vi "rma.vi"() -> ()   [LabVIEW 2016]
panel:
  out "new picture":picture
  out "Waveform Chart":cluster{"xpp":dbl, "SP":dbl}(graph)
  in  "Stop Button":bool
  in  "Ki":dbl
  in  "KD":dbl
  in  "kP":dbl
  in  "SP":dbl
  in  "F":dbl
  in  "k":dbl
  in  "b":dbl
  in  "m":dbl
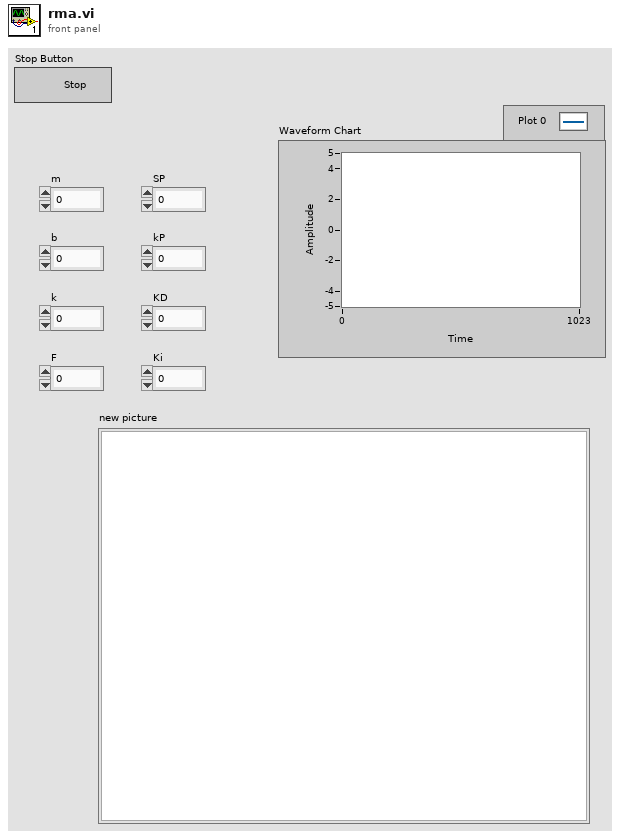
[diagram p1: front panel]
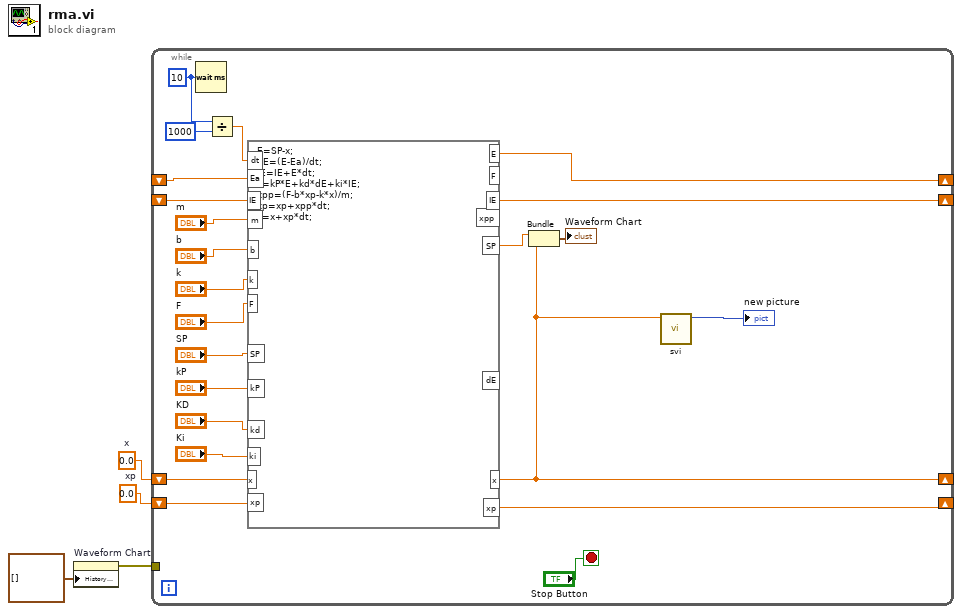
[diagram p0: block diagram]
diagram:
  w3 = 0.0  # xp
  w4 = 0.0  # x
  n1 = property on="Waveform Chart" class="WFChart (strict)"("History Data"=cluster{"xpp":dbl, "SP":dbl}[] []) -> (error out=w1:errorcluster)  [unwired: 2 in, 1 out]
  n2 = while {
    shift-right: [w5] -> _
    shift-left: w4 -> [w21]
    shift-right: [w20] -> _
    shift-left: w3 -> [w22]
    tunnel: w1 -> [_]
    shift-right: [w10] -> _
    shift-left: _ -> [w9]
    shift-right: [w8] -> _
    shift-left: _ -> [w7]
    stop <- "Stop Button" stop-if-true
    w19 = u32 10 ("milliseconds to wait")
    n3 = Wait (ms)(milliseconds to wait=w19) -> ()  [unwired: 1 out]
    n4 = Divide(x=w19, y=u32 1000) -> (x/y=w17:dbl)
    n5 = formula code="E=SP-x;\ndE=(E-Ea)/dt;\nIE=IE+E*dt;\nF=kP*E+kd*dE+ki*IE;\nxpp=(F-b*xp-k*x)/m;\nxp=xp+xpp*dt;\nx=x+xp*dt;"("m"="m", "b"="b", "k"="k", "F"="F", "x"=w21, "xp"=w22, "dt"=w17, "SP"="SP", "kP"="kP", "kd"="KD", "ki"="Ki", "Ea"=w9, "IE"=w7) -> ("x"=w5:dbl, "xp"=w20:dbl, "E"=w10:dbl, "SP"=w13:dbl, "IE"=w8:dbl)  [unwired: 3 out]
    n6 = Bundle("SP"=w13, "x"=w5) -> (→"Waveform Chart":cluster{"SP":dbl, "x":dbl})  [unwired: 1 in]
    n7 = call "svi.vi"("x"=w5) -> ("new picture"=→"new picture":picture)  [unwired: 10 in]
  }
